vi "Initialize.vi"(8 "error in (no error)":errorcluster, 9 "Requestor":string, 10 "Requestee":string, 11 "Mag Lab Hardware in":refnum<class "Keithley Meter.lvclass">) -> (0 "error out":errorcluster, 3 "Mag Lab Hardware out":refnum<class "Keithley Meter.lvclass">)   [LabVIEW 2015, in "Keithley Meter.lvclass"]
uses:
  Keithley Meter.lvclass
  NHMFL_Core/Libraries/Instruments/Keithley/Meter/Keithley Meter Parameters.ctl
  NHMFL_Core/Libraries/Instruments/Keithley/Meter/KeithleyMeter Function.ctl
  Mag Lab Hardware.lvclass/Mag Lab Hardware.ctl
  Keithley Meter.lvclass/Keithley Meter.ctl
  NHMFL_Core/Libraries/Instruments/GPIB/VISA  Send Receive.vi
  Meter/Meter.lvclass
  Mag Lab Properties/Mag Lab Parameters.lvclass
  Mag Lab Hardware.lvclass
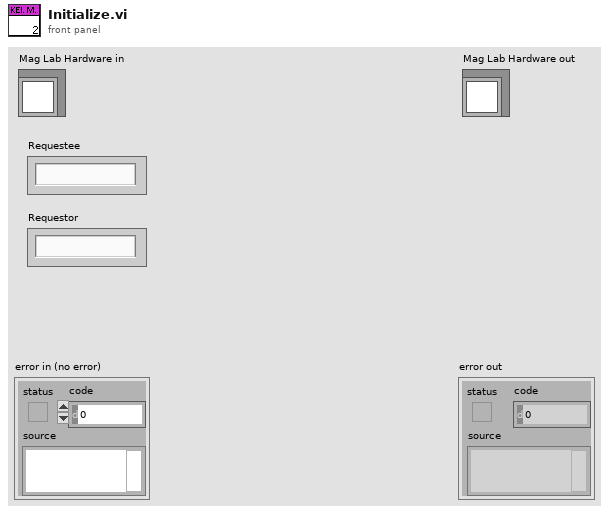
[diagram p1: front panel]
types:
  T1 = typedef "Keithley Meter Parameters.ctl" = cluster{"Range (-1: auto)":dbl, "Integration Time (NPLCs)":dbl, "Function":T2, "W Offset comp":bool, "4-wire W":bool, "Scale":dbl, "Offset":dbl}
  T2 = typedef "KeithleyMeter Function.ctl" = enum16{"VOLTAGE", "CURRENT", "RESISTANCE"}
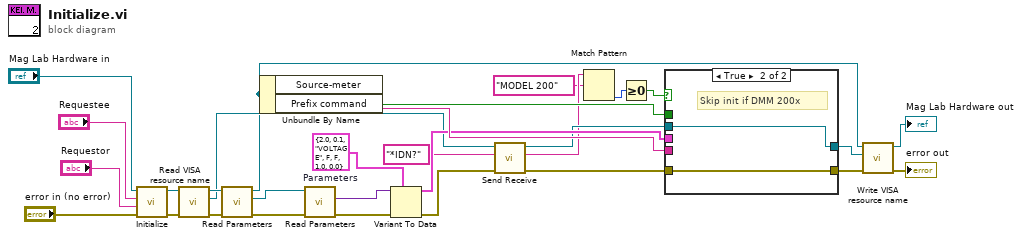
[diagram p0: block diagram]
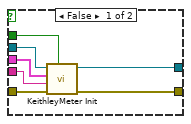
[diagram p2: hidden frame]
diagram:
  w17 = T1 {"Range (-1: auto)"=2.0, "Integration Time (NPLCs)"=0.1, "Function"=enum."VOLTAGE", "W Offset comp"=FALSE, "4-wire W"=FALSE, "Scale"=1.0, "Offset"=0.0}  # Parameters
  n1 = call-parent "Initialize.vi"("error in (no error)"="error in (no error)", "Requestor"="Requestor", "Requestee"="Requestee", "Mag Lab Root in"="Mag Lab Hardware in") -> ("error out"=w22:errorcluster, "Mag Lab Root out"=w26:refnum<class "Keithley Meter.lvclass">)  [unwired: 6 in]
  n2 = call "Read VISA resource name.vi"("error in (no error)"=w22, "Mag Lab Hardware in"=w26) -> ("error out"=w16:errorcluster, "VISA resource name"=w9:refnum<visa-resource-name>, "Mag Lab Hardware out"=w18:refnum<class "Keithley Meter.lvclass">)  [unwired: 7 in]
  n3 = call-dynamic "Read Parameters.vi"("error in (no error)"=w16, "Mag Lab Root in"=w18) -> ("error out"=w13:errorcluster, "Mag Lab Parameters.lvclass"=w15:refnum<class "Mag Lab Parameters.lvclass">, "Mag Lab Root out"=w1:refnum<class "Keithley Meter.lvclass">)  [unwired: 7 in]
  n4 = Unbundle By Name(w1) -> ("Source-meter"=w25:bool, "Prefix command"=w24:string)
  n5 = call-dynamic "Read Parameters.vi"("error in (no error)"=w13, "Mag Lab Parameters in"=w15) -> ("error out"=w12:errorcluster, "Parameters"=w14:variant)  [unwired: 7 in, 1 out]
  n6 = Variant To Data(error in=w12, type=w17, Variant=w14) -> (data=w11:T1, error out=w10:errorcluster)
  n7 = call-poly "Send Receive.vi"("error in (no error)"=w10, "data string in"="*IDN?", "VISA Resource Name"=w9) -> ("error out"=w7:errorcluster, "data string out"=w6:string, "VISA Resource Name Out"=w8:refnum<visa-resource-name>)  [unwired: 6 in]
  n8 = Match Pattern(string=w6, regular expression="MODEL 200") -> (offset past match=w4:i32)  [unwired: 1 in, 3 out]
  n9 = Greater Or Equal To 0?(x=w4) -> (x >= 0?=w2:bool)
  n10 = case shown="True" w2 {
    tunnel: w25 -> [w37 _]
    tunnel: w24 -> [w36 _]
    tunnel: [w35 w38] -> w23
    tunnel: [w34 w39] -> w21
    tunnel: w11 -> [w33 _]
    tunnel: w8 -> [w32 w38]
    tunnel: w7 -> [w31 w39]
    frame False {
      n11 = call "KeithleyMeter Init.vi"("Source-meter"=w37, "Error In"=w31, "Prefix command"=w36, "Parameters"=w33, "VISA resource name"=w32) -> ("Error Out"=w34:errorcluster, "VISA resource name out"=w35:refnum<visa-resource-name>)  [unwired: 5 in]
    }
    frame True {
      # "Skip init if DMM 200x"
    }
  }
  n12 = call "Write VISA resource name.vi"("error in (no error)"=w21, "VISA resource name"=w23, "Mag Lab Hardware in"=w1) -> ("error out"=→"error out":errorcluster, "Mag Lab Hardware out"=→"Mag Lab Hardware out":refnum<class "Keithley Meter.lvclass">)  [unwired: 7 in]
